vi "UI History Build Test Details.vi"(9 "index (row)":i32, 11 "Array":string[][](array[string])) -> (3 "Value":T1)   [LabVIEW 2020]
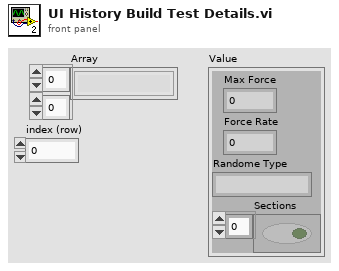
[diagram p1: front panel]
types:
  T1 = cluster{"Max Force":dbl, "Force Rate":dbl, "Randome Type":string, "Sections":bool[]}
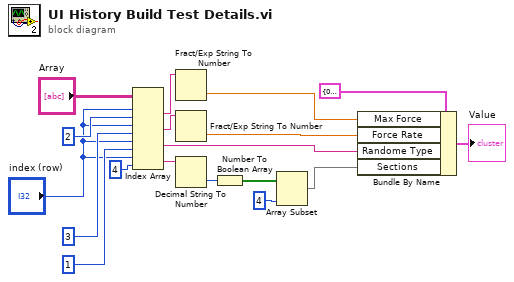
[diagram p0: block diagram]
diagram:
  n1 = Index Array(array="Array", index (row) #1="index (row)", index (col) #1=2 ("disabled index (col)"), index (row) #2="index (row)", index (col) #2=3 ("disabled index (col)"), index (row) #3="index (row)", index (col) #3=1 ("disabled index (col)"), index (row) #4="index (row)", index (col) #4=4 ("disabled index (col)")) -> (element #1=w6:string, element #2=w8:string, element #3=w12:string, element #4=w14:string)
  n2 = Fract/Exp String To Number(string=w6) -> (number=w7:dbl)  [unwired: 3 in, 1 out]
  n3 = Fract/Exp String To Number(string=w8) -> (number=w10:dbl)  [unwired: 3 in, 1 out]
  n4 = Decimal String To Number(string=w14) -> (number=w15:i32)  [unwired: 2 in, 1 out]
  n5 = Number To Boolean Array(number=w15) -> (Boolean array=w16:bool[])
  n6 = Array Subset(array=w16, length=4) -> (w17:bool[])  [unwired: 1 in]
  n7 = Bundle By Name(cluster=T1 {"Max Force"=0.0, "Force Rate"=0.0, "Randome Type"="", "Sections"=[]} ("Value"), "Max Force"=w7, "Force Rate"=w10, "Randome Type"=w12, "Sections"=w17) -> (→"Value":T1)
